vi "main.vi"() -> ()   [LabVIEW 2021]
panel:
  out "Filtration (mg/cm^2)":dbl
  in  "Density (g/cm^3)":dbl
  in  "Thickness (mm)":dbl
  out "Thickness (mm)":dbl
  in  "Densitiy (g/cm^3)":dbl
  in  "Filtration (mg/cm^2)":dbl
  # "Cálculo de espesor dada una filtración"
  # "Cálculo de fitlración por espesor de material y densidad"
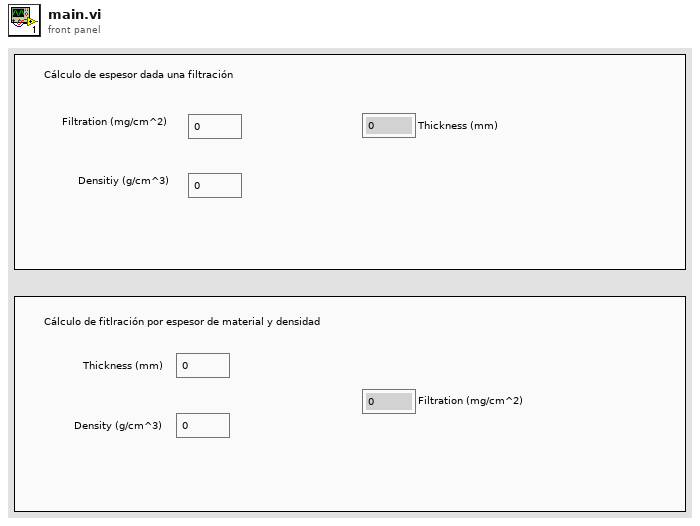
[diagram p1: front panel]
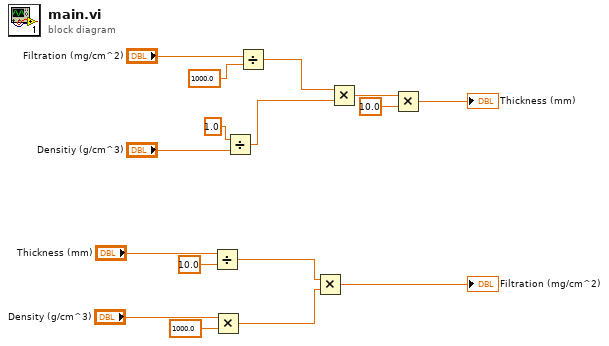
[diagram p0: block diagram]
diagram:
  n1 = Divide(x="Thickness (mm)", y=10.0) -> (x/y=w3:dbl)
  n2 = Multiply(x="Density (g/cm^3)", y=1000.0) -> (x*y=w2:dbl)
  n3 = Divide(x=1.0, y="Densitiy (g/cm^3)") -> (x/y=w15:dbl)
  n4 = Divide(x="Filtration (mg/cm^2)", y=1000.0) -> (x/y=w14:dbl)
  n5 = Multiply(x=w3, y=w2) -> (x*y=→"Filtration (mg/cm^2)":dbl)
  n6 = Multiply(x=w14, y=w15) -> (x*y=w10:dbl)
  n7 = Multiply(x=w10, y=10.0) -> (x*y=→"Thickness (mm)":dbl)
